vi "DtCreateCtrTwoEdgeChan.vi"(1 "Start Edge":i32(ring)=752 items=["GateRising"=750, "GateFalling"=751, "ClockRising"=752, "ClockFalling"=753], 2 "Stop Edge":i32(ring)=752 items=["GateRising"=750, "GateFalling"=751, "ClockRising"=752, "ClockFalling"=753], 5 "Board Name":string, 7 "Counter Num":u32, 11 "error in (no error)":errorcluster) -> (4 "Task out":i32, 15 "error out":errorcluster)   [LabVIEW 2016]
doc: "Creates one or more virtual counter/timer channels that measure the time, in milliseconds, between a specified start edge and stop edge of the counter's clock or gate input signal, and then stops.\n\nThe start edge and the stop edge can occur on the rising edge of the gate input signal, the falling edge of the gate input signal, the rising edge of the clock input signal, or the falling edge of the clock input signal.\n\nThis type of task is also called edge-to-edge measurement. To use this VI, your device must support edge-to-edge measurement mode.\n\nOnce you have created a virtual counter/timer channel for an edge-to-edge measurement task, you can start the task and read the measurement using the DtOLRead (Read Single Channel - Single Sample) VI. Note that if you read the counter/timer before the measurement is complete, 0 is returned.\n\nTo read another value, you must first restart the task using the ReStart VI. If you want the edge-to-edge measurement to restart automatically, use the DtOLCreateTask (Counter Input - Cont Measure) VI instead."
uses:
  <userlib>/LV-Link3/DtLvLink.lvlib
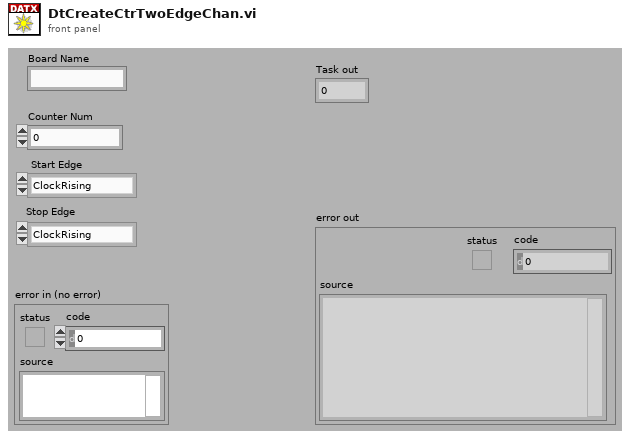
[diagram p1: front panel]
types:
  T1 = enum32{"AnalogInput", "AnalogOutput", "DigitalInput", "DigitalOutput", "Quadrature", "CounterTimer"}
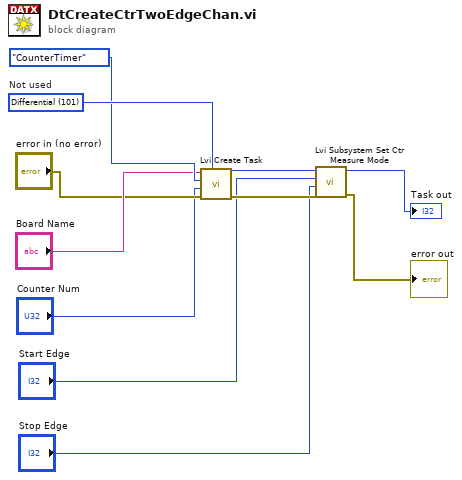
[diagram p0: block diagram]
diagram:
  w11 = 101 items=["SingleEnded"=100, "Differential"=101]  # Not used
  n1 = call <userlib>:"Lvi Create Task.vi"("SEorDiff"=w11, "error in (no error)"="error in (no error)", "SubSysIndex"="Counter Num", "ChanType"=T1."CounterTimer", "BoardName"="Board Name") -> ("error out"=w5:errorcluster, "TaskRef"=w6:i32)  [unwired: 4 in, 1 out]
  n2 = call <userlib>:"Lvi Subsystem Set Ctr Measure Mode.vi"("error in (no error)"=w5, "StopEdge"="Stop Edge", "StartEdge"="Start Edge", "TaskRef"=w6) -> ("error out"=→"error out":errorcluster, "TaskRef out"=→"Task out":i32)  [unwired: 5 in, 1 out]
